vi "Radians to Degrees (Scalar EXT).vi"(3 "angle (rad)":ext) -> (1 "angle (deg)":ext)   [LabVIEW 2017, in "NI_AngleManipulation.lvlib"]
doc: "Converts an angle from radians to degrees."
uses:
  <vilib>/Utility/AngleManip/NI_AngleManipulation.lvlib
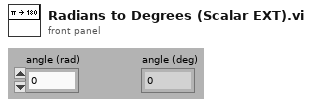
[diagram p1: front panel]
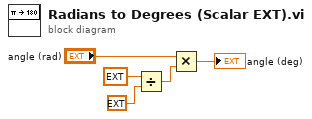
[diagram p0: block diagram]
diagram:
  n1 = Divide(x=ext 180.0 ("y"), y=ext 3.1415926535897932385) -> (x/y=w2:ext)
  n2 = Multiply(x="angle (rad)", y=w2) -> (x*y=→"angle (deg)":ext)
